vi "运维调试_氨氮.vi"() -> ()   [LabVIEW 2016, in "斯坦道氨氮.lvlib"]
uses:
  <vilib>/Utility/miscctls.llb/LVPointTypeDef.ctl
  <vilib>/Utility/config.llb/NI_LVConfig.lvlib
panel:
  in  "模块启用":bool
  in  "串口设置":bool
  in  "备用系数一键写入":bool
  in  "公式一键写入":bool
  in  "流程文件路径":path=path "C:/Users/std/Documents/斯坦道流程文件/流程.xml"
  in  "曲线模型":cluster{"X^2":dbl, "X":dbl, "B":dbl}(xcontrol)
  in  "质控参数设置":bool
  out "字符串":string
  in  "氨氮自动测试量程配置":T1
  out "ADC":sgl
  out "温度2":sgl
  out "温度1":sgl
  out "固件版本号":string
  in  "数组":string[](array[string])
  in  "备用系数写入":bool
  in  "备用系数读取":bool
  in  "备用系数":T2
  in  "量程切换阈值写入":bool
  in  "量程切换阈值读取":bool
  in  "量程切换阈值":cluster{"阈值":dbl, "标液浓度":dbl}
  in  "参数下拉列表":enum16{"氨氮", "总磷"}(ring)
  in  "量程下拉列表":enum16{"低量程", "高量程"}(ring)
  in  "测量模式下拉列表":enum16{"水样测量", "空白核查", "跨度核查", "标样核查", "加标回收"}(ring)
  in  "公式":cluster{"X^2":dbl, "X":dbl, "b":dbl}
  in  "写公式":bool
  in  "读公式":bool
  in  "返回":bool
  in  "设置":bool
  out "序列号":string="序列号"
  out "氨氮测量数据":T3(xcontrol)
  out "集成报警信息":string
  out "定时启动":bool
  out "总磷总氮运行状态":T4(xcontrol)
  in  "停止":bool
  in  "手动启动":bool
  in  "单步测试":bool
  in  "总磷氨氮调试":u16[](xcontrol)
  out "F3":sgl format="%#.6f"
  out "F2":sgl format="%#.6f"
  out "F1":sgl format="%#.6f"
  out "F0":sgl format="%#.6f"
  out "多列列表框":i32(listbox)
  # "参数设置"
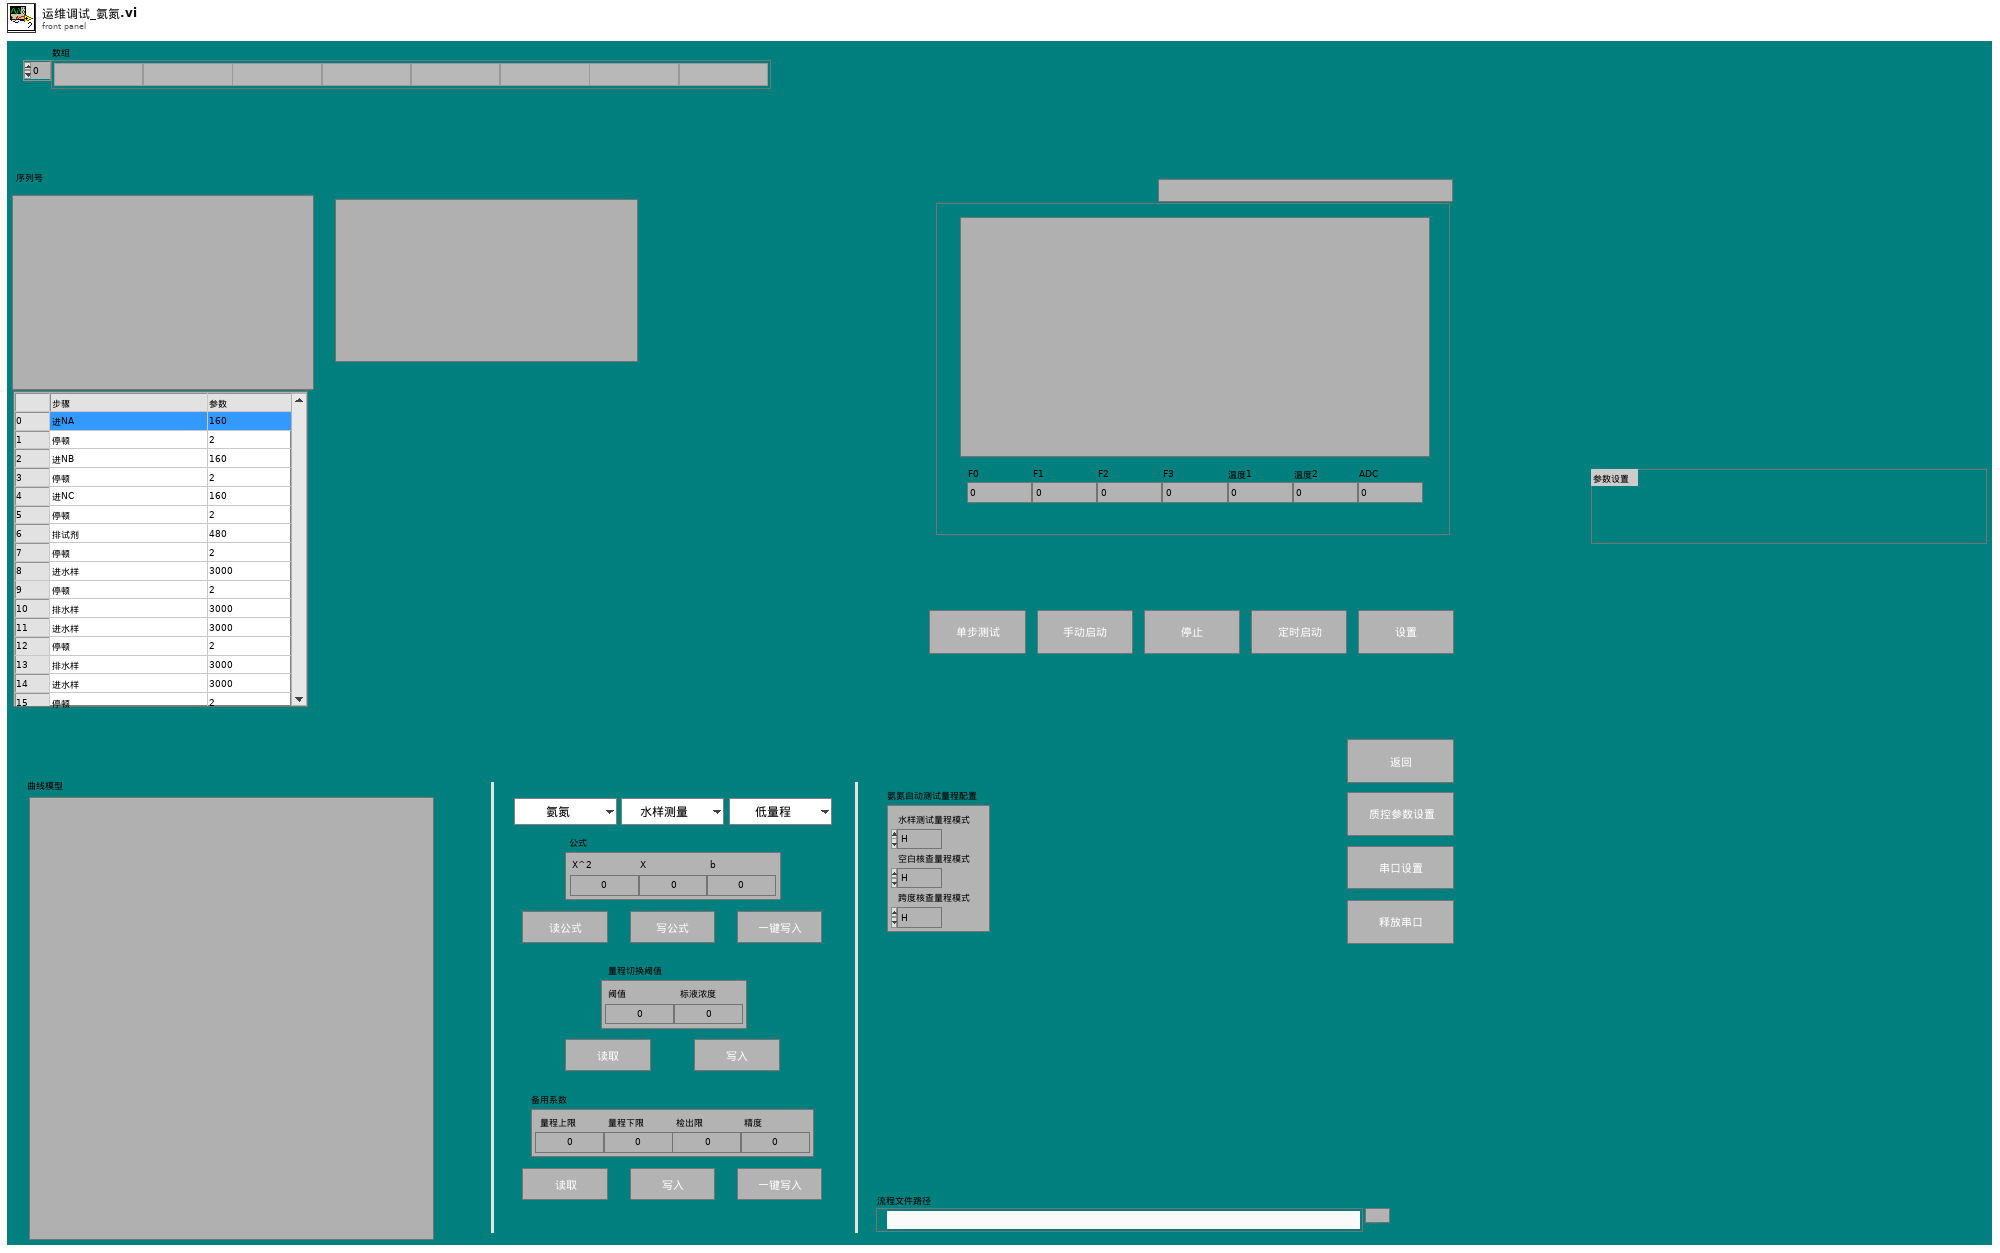
[diagram p1: front panel]
types:
  T1 = cluster{"水样测试量程模式":enum16{"H", "L", "AUTO"}, "空白核查量程模式":enum16{"H", "L", "AUTO"}, "跨度核查量程模式":enum16{"H", "L", "AUTO"}}
  T2 = cluster{"量程上限":dbl, "量程下限":dbl, "检出限":dbl, "精度":dbl}
  T3 = cluster{"flowid":u16, "测量精度":u16, "测量数据区":cluster{"因子编码":u32, "单位":u16, "标样参考值":sgl, "水样数据时间":timestamp, "水样实测值":sgl, "水样数据标识":string, "标样数据时间":timestamp, "标样实测值":sgl, "标样数据标识":string, "空白数据时间":timestamp, "空白实测值":sgl, "空白数据标识":string, "零点核查数据时间":timestamp, "零点核查实测值":sgl, "零点核查数据标识":string, "跨度核查数据时间":timestamp, "跨度核查实测值":sgl, "跨度核查数据标识":string, "加标回收数据时间":timestamp, "加标回收实测值":sgl, "加标回收数据标识":string, "平行样数据时间":timestamp, "平行样实测值":sgl, "平行样数据标识":string}}
  T4 = cluster{"系统时间":timestamp, "工作状态":enum16{"空闲", "水样测试", "标样核查", "零点核查", "跨度核查", "空白测试", "平行样测试", "加标回收", "空白校准", "标样校准", "初始化（清洗）"}, "测量模式":enum16{"待机", "连续模式", "周期模式", "定点模式", "受控模式", "手动模式"}, "告警代码":enum16{"无告警", "缺试剂告警", "缺水样告警", "缺蒸馏水告警", "缺标液告警", "仪表漏液告警", "标定异常告警", "超量程告警", "加热异常", "低试剂预警", "超上限告警", "超下限告警", "仪表内部其他异常", "滴定异常告警", "电极异常告警", "量程切换告警", "参数设置告警", "PH电极电位异常", "电导率电极异常", "浊度光度异常", "溶解氧电极异常", "溶解氧光强异常", "温度异常告警", "PH异常告警", "溶解氧异常告警", "电导率异常告警", "浊度异常告警", "叶绿素异常告警", "藻密度异常告警", "蓝绿藻异常告警", "ORP异常告警", "氨氮异常告警", "清洁刷异常告警", "SD卡异常告警", "蓝牙异常告警", "Wifi异常告警", "流程异常告警"}, "故障代码":enum16{"无故障", "电机故障", "温度故障", "通讯故障", "滴定故障"}, "日志代码":u16, "软件版本":u16, "F0":sgl, "F1":sgl, "F2":sgl, "F3":sgl, "T":sgl, "H":sgl, "id":u16, "flowid":u16, "量程":u16, "总磷控温温度1":sgl, "营养盐控温温度2":sgl, "ADC":sgl}
  T5 = enum16{"启动测量", "标样核查", "零点核查", "跨度核查", "空白测试", "平行样测试", "加标回收", "空白校准", "标样校准", "初始化（清洗）", "停止测试", "仪器重启", "校时", "模式设置", "测量间隔设置"}
  T6 = cluster{"控制命令":enum16{"启动测量", "标样核查", "零点核查", "跨度核查", "空白测试", "平行样测试", "加标回收", "空白校准", "标样校准", "初始化（清洗）", "停止测试", "仪器重启", "校时", "模式设置", "测量间隔设置"}, "周期设置类型":enum16{"定点启动", "间隔启动"}, "定时功能启用":bool, "定时间隔":dbl, "24H周期设置":bool[], "空白核查时间":u16, "跨度核查时间":u16, "质控频次":enum16{"关闭", "每天", "星期一", "星期二", "星期三", "星期四", "星期五", "星期六", "星期日"}}
  T7 = enum16{"关闭", "每天", "星期一", "星期二", "星期三", "星期四", "星期五", "星期六", "星期日"}
  T8 = enum32{"Bad", "Idle", "Run top level", "Running"}
  T9 = typedef "LVDateTimeRec.ctl" = cluster{"秒数的小数部分":dbl, "秒":i32, "分":i32, "时":i32, "日":i32, "月":i32, "年":i32, "天数（周）":i32, "天数（年）":i32, "DST":i32}
  T10 = typedef "LVPointTypeDef.ctl" = cluster{"Horizontal":i16, "Vertical":i16}
  T11 = cluster{"因子编码":u32, "单位":u16, "标样参考值":sgl, "水样数据时间":timestamp, "水样实测值":sgl, "水样数据标识":string, "标样数据时间":timestamp, "标样实测值":sgl, "标样数据标识":string, "空白数据时间":timestamp, "空白实测值":sgl, "空白数据标识":string, "零点核查数据时间":timestamp, "零点核查实测值":sgl, "零点核查数据标识":string, "跨度核查数据时间":timestamp, "跨度核查实测值":sgl, "跨度核查数据标识":string, "加标回收数据时间":timestamp, "加标回收实测值":sgl, "加标回收数据标识":string, "平行样数据时间":timestamp, "平行样实测值":sgl, "平行样数据标识":string}
  T12 = enum16{"空闲", "水样测试", "标样核查", "零点核查", "跨度核查", "空白测试", "平行样测试", "加标回收", "空白校准", "标样校准", "初始化（清洗）"}
  T13 = cluster{"启动模式":enum16{"跨度核查", "水样测量", "空白核查", "标样核查", "加标回收"}, "启动参数":u16, "量程":enum16{"低量程", "高量程"}}
  T14 = cluster{"时间标识":timestamp, "设备":string, "日志信息":string, "流程参数":string}
  T15 = cluster{"时间标识":timestamp, "设备":string, "日志信息":string}
  T16 = enum16{"无告警", "缺试剂告警", "缺水样告警", "缺蒸馏水告警", "缺标液告警", "仪表漏液告警", "标定异常告警", "超量程告警", "加热异常", "低试剂预警", "超上限告警", "超下限告警", "仪表内部其他异常", "滴定异常告警", "电极异常告警", "量程切换告警", "参数设置告警", "PH电极电位异常", "电导率电极异常", "浊度光度异常", "溶解氧电极异常", "溶解氧光强异常", "温度异常告警", "PH异常告警", "溶解氧异常告警", "电导率异常告警", "浊度异常告警", "叶绿素异常告警", "藻密度异常告警", "蓝绿藻异常告警", "ORP异常告警", "氨氮异常告警", "清洁刷异常告警", "SD卡异常告警", "蓝牙异常告警", "Wifi异常告警", "流程异常告警"}
  T17 = typedef "LVRowAndColumnUnsignedTypeDef.ctl" = cluster{"Row":u32, "Column":u32}
  T18 = typedef "NI_LVConfig.lvlib/Config Data RefNum.ctl" = refnum<k1>
  T19 = cluster{"站号":u16, "量程切换":enum32{"H", "L", "AUTO"}, "控制命令":enum16{"启动测量", "标样核查", "零点核查", "跨度核查", "空白测试", "平行样测试", "加标回收", "空白校准", "标样校准", "初始化（清洗）", "停止测试", "仪器重启", "校时", "模式设置", "测量间隔设置"}, "模式设置":enum16{"待机", "连续模式", "周期模式", "定点模式", "受控模式", "手动模式"}, "测量间隔":u16}
  T20 = cluster{"跨度值":dbl, "零点标准液浓度":dbl, "跨度标准液浓度":dbl, "标准液标准浓度":dbl}
  T21 = cluster{"确定":bool, "跨度值":dbl, "零点标准液浓度":dbl, "跨度标准液浓度":dbl, "标准液标准浓度":dbl}
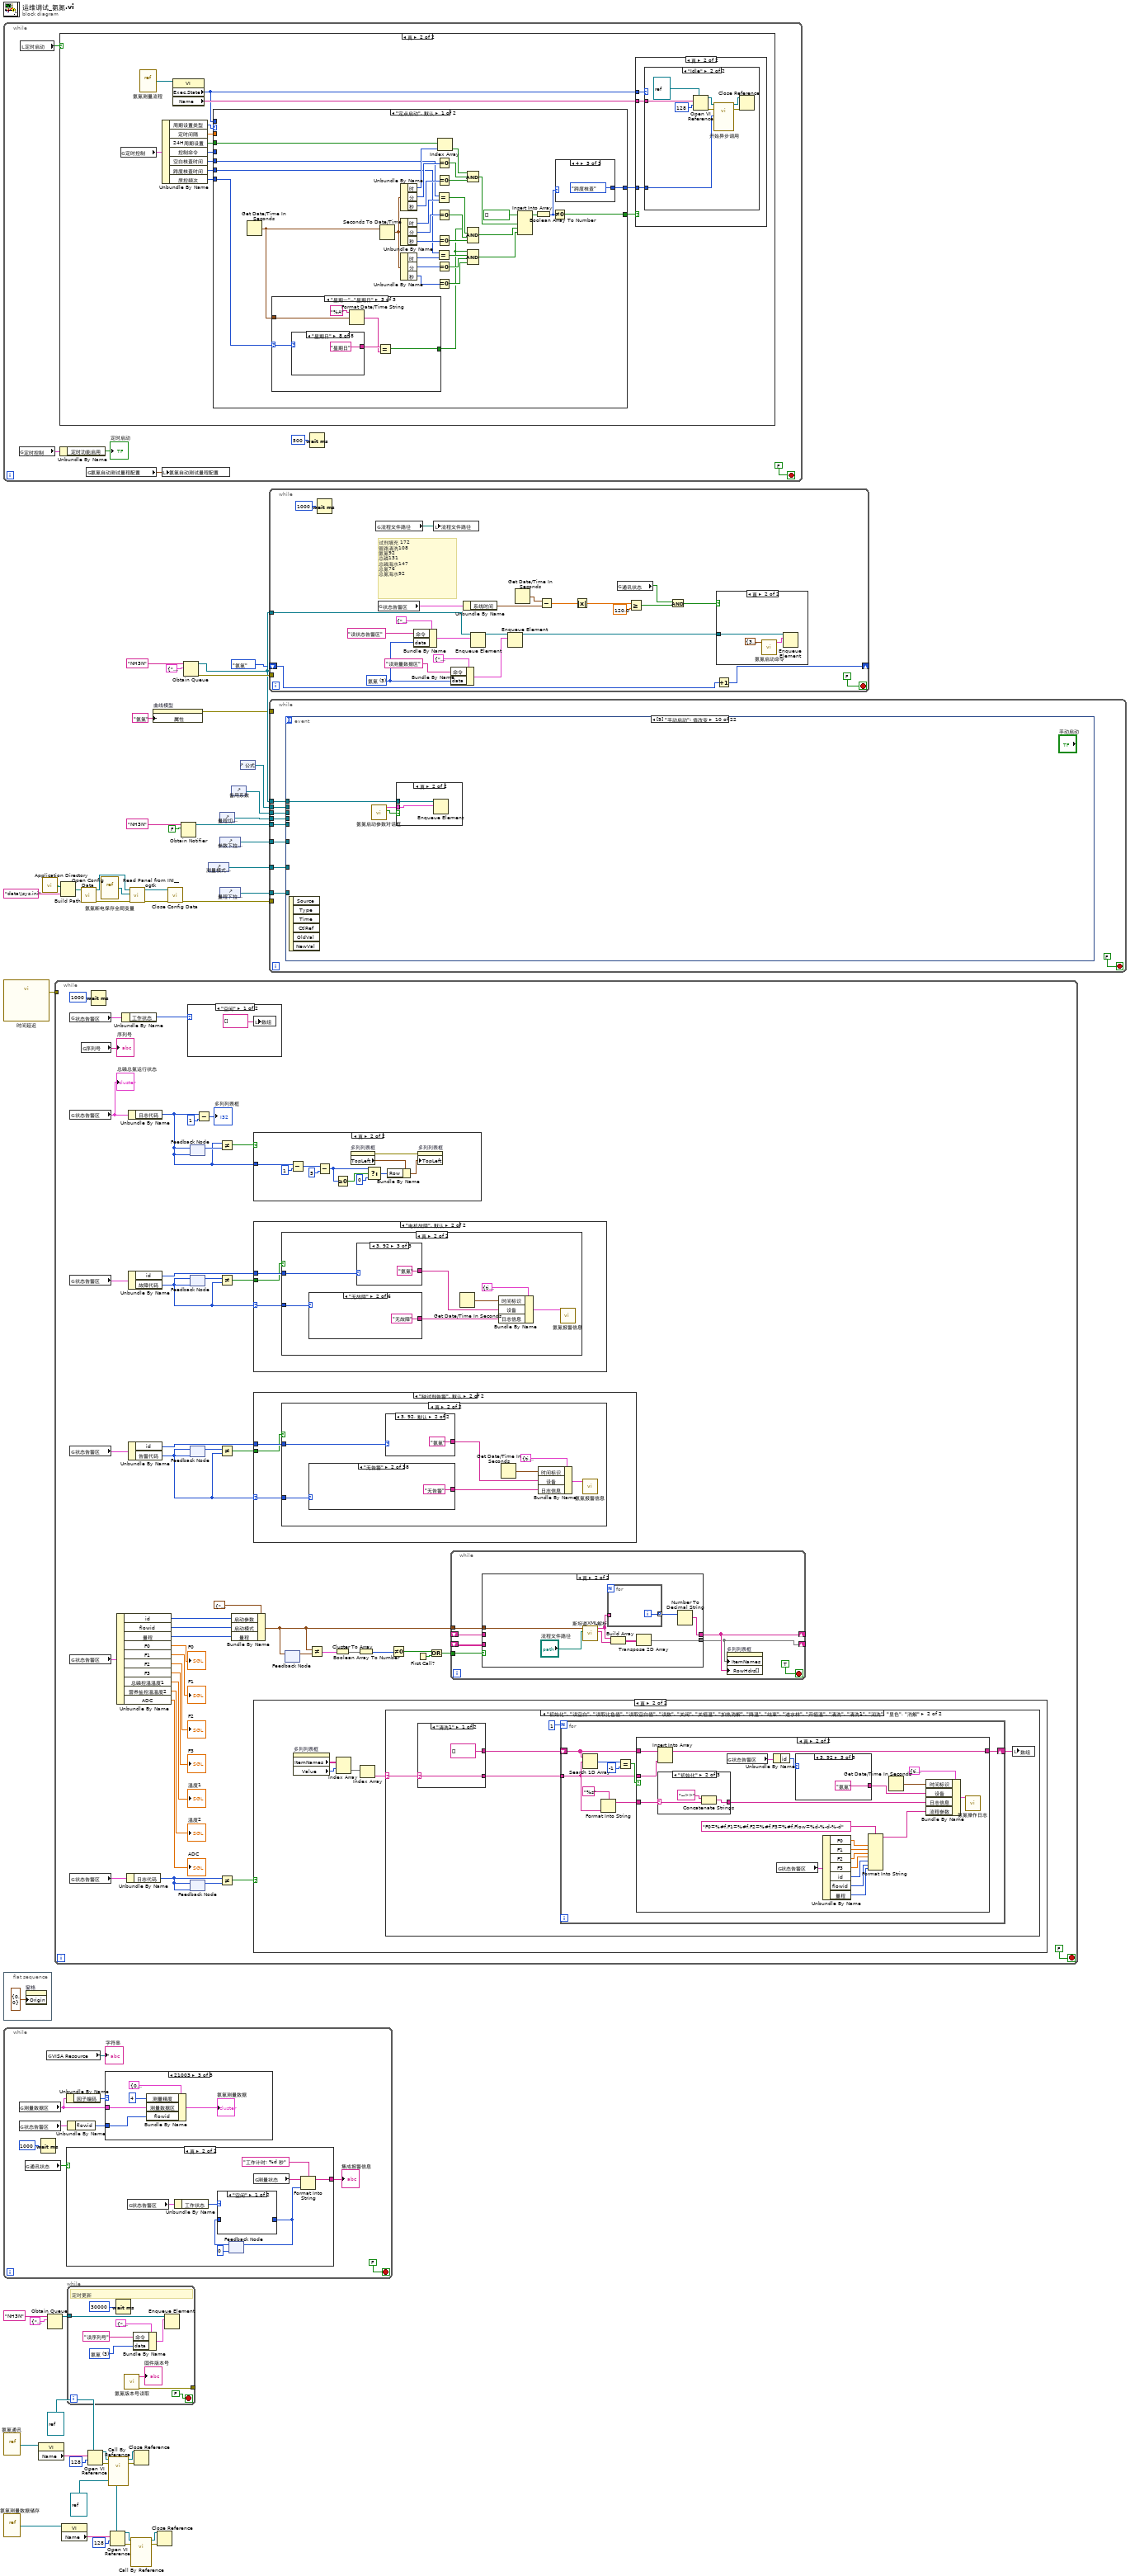
[diagram p0: block diagram]
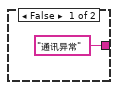
[diagram p2: hidden frame]
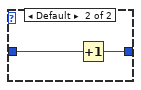
[diagram p3: hidden frame]
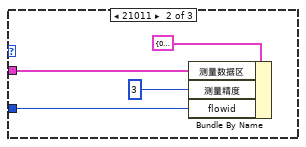
[diagram p5: hidden frame]
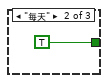
[diagram p8: hidden frame]
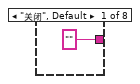
[diagram p9: hidden frame]
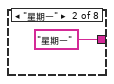
[diagram p10: hidden frame]
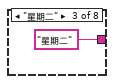
[diagram p11: hidden frame]
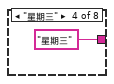
[diagram p12: hidden frame]
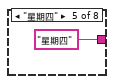
[diagram p13: hidden frame]
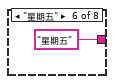
[diagram p14: hidden frame]
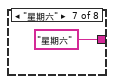
[diagram p15: hidden frame]
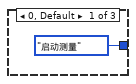
[diagram p16: hidden frame]
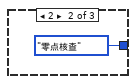
[diagram p17: hidden frame]
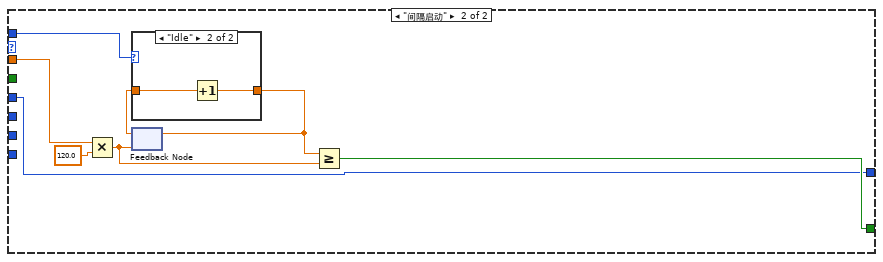
[diagram p18: hidden frame]
diagram:
  n1 = while {
    stop <- FALSE stop-if-true
    n2 = global read "氨氮断电保存全局变量.vi" "定时控制"() -> (w48:T6)
    n3 = local read "定时启动"() -> (w49:bool)
    n4 = case shown="真" w49 {
      frame False {
      }
      frame True {
        n5 = global read "氨氮断电保存全局变量.vi" "定时控制"() -> (w64:T6)
        n6 = vi-ref "氨氮测量流程.vi"() -> (w63:refnum<vi>)
        n7 = Unbundle By Name(w64) -> ("周期设置类型"=w60:enum16{"定点启动", "间隔启动"}, "定时间隔"=w59:dbl, "24H周期设置"=w58:bool[], "控制命令"=w57:T5, "空白核查时间"=w54:u16, "跨度核查时间"=w53:u16, "质控频次"=w52:T7)
        n8 = property class="VI"(reference=w63) -> ("Exec.State"=w61:T8, "Name"=w62:string)  [unwired: 1 in, 2 out]
        n9 = case shown="\"定点启动\", 默认" w60 {
          tunnel: w59 -> [_ w120]
          tunnel: w58 -> [w88 _]
          tunnel: w61 -> [_ w123]
          tunnel: [w66 w118] -> w55
          tunnel: w57 -> [_ w116]
          tunnel: [w92 w116] -> w56
          tunnel: w52 -> [w91 _]
          tunnel: w54 -> [w84 _]
          tunnel: w53 -> [w73 _]
          frame "定点启动", Default {
            n10 = Get Date/Time In Seconds() -> (seconds since 1Jan1904=w90:timestamp)
            n11 = case shown="\"星期一\"..\"星期日\"" w91 {
              selector: w91 -> [_ _ w102]
              tunnel: w90 -> [_ _ w103]
              tunnel: [_ TRUE w99] -> w72
              frame "关闭", Default {
              }
              frame "每天" {
              }
              frame "星期一".."星期日" {
                n12 = case shown="\"星期日\"" w102 {
                  tunnel: ["" ("时间格式字符串(%c)") "星期一" ("时间格式字符串(%c)") "星期二" ("时间格式字符串(%c)") "星期三" ("时间格式字符串(%c)") "星期四" ("时间格式字符串(%c)") "星期五" ("时间格式字符串(%c)") "星期六" ("时间格式字符串(%c)") "星期日" ("时间格式字符串(%c)")] -> w101
                  frame "关闭", Default {
                  }
                  frame "星期一" {
                  }
                  frame "星期二" {
                  }
                  frame "星期三" {
                  }
                  frame "星期四" {
                  }
                  frame "星期五" {
                  }
                  frame "星期六" {
                  }
                  frame "星期日" {
                  }
                }
                n13 = Format Date/Time String(time format string (%c)="%A" ("时间格式字符串(%c)"), seconds (now)=w103) -> (date/time string=w100:string)  [unwired: 1 in]
                n14 = Equal?(x=w101, y=w100) -> (x = y?=w99:bool)
              }
            }
            n15 = Seconds To Date/Time(time stamp (now)=w90) -> (date time rec=w74:T9)  [unwired: 1 in]
            n16 = Unbundle By Name(w74) -> ("时"=w97:i32, "分"=w95:i32, "秒"=w96:i32)
            n17 = Unbundle By Name(w74) -> ("时"=w85:i32, "分"=w87:i32, "秒"=w86:i32)
            n18 = Unbundle By Name(w74) -> ("时"=w77:i32, "分"=w75:i32, "秒"=w76:i32)
            n19 = Equal?(x=w84, y=w85) -> (x = y?=w83:bool)
            n20 = Equal?(x=w73, y=w77) -> (x = y?=w78:bool)
            n21 = Equal To 0?(x=w95) -> (x = 0?=w94:bool)
            n22 = Equal To 0?(x=w96) -> (x = 0?=w93:bool)
            n23 = Equal To 0?(x=w87) -> (x = 0?=w82:bool)
            n24 = Equal To 0?(x=w86) -> (x = 0?=w81:bool)
            n25 = Equal To 0?(x=w75) -> (x = 0?=w79:bool)
            n26 = Equal To 0?(x=w76) -> (x = 0?=w80:bool)
            n27 = Index Array(array=w88, index=w97) -> (element=w89:bool)
            n28 = Compound Arithmetic op=AND ("复合运算")(w89, w94, w93) -> (w70:bool)
            n29 = Compound Arithmetic op=AND ("复合运算")(w72, w83, w82, w81) -> (w69:bool)
            n30 = Compound Arithmetic op=AND ("复合运算")(w72, w78, w79, w80) -> (w68:bool)
            n31 = Insert Into Array(array=bool[] [], new element #1=w70, new element #2=w69, new element #3=w68) -> (w67:bool[])  [unwired: 1 in]
            n32 = Boolean Array To Number(Boolean array=w67) -> (number=w65:u32)
            n33 = Not Equal To 0?(x=w65) -> (x != 0?=w66:bool)
            n34 = case shown="4" w65 {
              tunnel: [T5."启动测量" ("控制命令") T5."零点核查" ("控制命令") T5."跨度核查" ("控制命令")] -> w92
              frame 0, Default {
              }
              frame 2 {
              }
              frame 4 {
              }
            }
          }
          frame "间隔启动" {
            n35 = Multiply(x=w120, y=120.0) -> (x*y=w117:dbl)
            n36 = feedback #1(w117) -> (w122:dbl)
            n37 = case shown="\"Idle\"" w123 {
              tunnel: w122 -> [_ w125]
              tunnel: [_ w124] -> w121
              frame "Bad", Default {
              }
              frame "Idle" {
                n38 = Increment(x=w125) -> (x+1=w124:dbl)
              }
            }
            n39 = feedback-in #1(w121) -> ()
            n40 = Greater Or Equal?(x=w121, y=w117) -> (x >= y?=w118:bool)
          }
        }
        n41 = case shown="真" w55 {
          tunnel: w62 -> [_ w128]
          tunnel: w56 -> [_ w127]
          tunnel: w61 -> [_ w126]
          frame False {
          }
          frame True {
            n42 = case shown="\"Idle\"" w126 {
              tunnel: w128 -> [_ w132]
              tunnel: w127 -> [_ w130]
              frame "Bad", Default {
              }
              frame "Idle" {
                n43 = Open VI Reference(type specifier VI Refnum (for type only)=refnum<vi> refnum, vi path=w132, options=128 ("选项")) -> (vi reference=w133:refnum<vi>, error out=w134:errorcluster)  [unwired: 3 in]
                n44 = call-by-ref "开始异步调用"(reference=w133, error in=w134, "控制命令"=w130) -> (reference out=w135:refnum<vi>, error out=w136:errorcluster)  [unwired: 11 in]
                n45 = Close Reference(reference=w135, error in (no error)=w136) -> ()  [unwired: 1 out]
              }
            }
          }
        }
      }
    }
    n46 = Unbundle By Name(w48) -> ("定时功能启用"=→"定时启动":bool)
    n47 = global read "氨氮断电保存全局变量.vi" "氨氮自动测试量程配置"() -> (w46:T1)
    n48 = local write "氨氮自动测试量程配置"(w46) -> ()
    n49 = Wait (ms)(milliseconds to wait=u32 500 ("等待时间（毫秒）")) -> ()  [unwired: 1 out]
  }
  n50 = call "时间延迟"() -> ("error out"=w18:errorcluster)  [unwired: 11 in]
  n51 = flat-sequence {
    frame #0 {
      n52 = property on="窗格" class="Pane"("Origin"=T10 {"Horizontal"=0, "Vertical"=0} ("原点")) -> ()  [unwired: 2 in, 2 out]
    }
  }
  n53 = while {
    stop <- FALSE stop-if-true
    n54 = global read "VAR氨氮全局变量.vi" "测量数据区"() -> (w144:T11)
    n55 = global read "VAR氨氮全局变量.vi" "状态告警区"() -> (w140:T4)
    n56 = global read "VAR氨氮全局变量.vi" "通讯状态"() -> (w142:bool)
    n57 = Wait (ms)(milliseconds to wait=u32 1000 ("等待时间（毫秒）")) -> ()  [unwired: 1 out]
    n58 = global read "氨氮断电保存全局变量.vi" "VISA Resource"() -> (→"字符串":refnum<visa-resource-name>)
    n59 = Unbundle By Name(w144) -> ("因子编码"=w143:u32)
    n60 = case shown="真" w142 {
      tunnel: ["通讯异常" ("集成报警信息") w149] -> w141
      frame False {
      }
      frame True {
        n61 = global read "VAR氨氮全局变量.vi" "状态告警区"() -> (w155:T4)
        n62 = Unbundle By Name(w155) -> ("工作状态"=w154:T12)
        n63 = feedback #2(0) -> (w152:i32)
        n64 = case shown="\"空闲\"" w154 {
          tunnel: w152 -> [_ w157]
          tunnel: [_ w156] -> w150
          frame "空闲" {
          }
          frame Default {
            n65 = Increment(x=w157) -> (x+1=w156:i32)
          }
        }
        n66 = feedback-in #2(w150) -> ()
        n67 = global read "VAR氨氮全局变量.vi" "测量状态"() -> (w148:string)
        n68 = Format Into String(format string="工作计时: %d 秒" ("格式字符串"), initial string=w148, w150) -> (resulting string=w149:string)  [unwired: 1 in, 1 out]
      }
    }
    "集成报警信息" <- w141
    n69 = Unbundle By Name(w140) -> ("flowid"=w139:u16)
    n70 = case shown="21003" w143 {
      tunnel: w144 -> [_ w161 w166]
      tunnel: w139 -> [_ w159 w164]
      frame Default {
      }
      frame 21011 {
        n71 = Bundle By Name(cluster=T3 {"flowid"=0, "测量精度"=0, "测量数据区"={"因子编码"=0, "单位"=0, "标样参考值"=0.0, "水样数据时间"=timestamp(0 s since 1904-01-01), "水样实测值"=0.0, "水样数据标识"="", "标样数据时间"=timestamp(0 s since 1904-01-01), "标样实测值"=0.0, "标样数据标识"="", "空白数据时间"=timestamp(0 s since 1904-01-01), "空白实测值"=0.0, "空白数据标识"="", "零点核查数据时间"=timestamp(0 s since 1904-01-01), "零点核查实测值"=0.0, "零点核查数据标识"="", "跨度核查数据时间"=timestamp(0 s since 1904-01-01), "跨度核查实测值"=0.0, "跨度核查数据标识"="", "加标回收数据时间"=timestamp(0 s since 1904-01-01), "加标回收实测值"=0.0, "加标回收数据标识"="", "平行样数据时间"=timestamp(0 s since 1904-01-01), "平行样实测值"=0.0, "平行样数据标识"=""}} ("氨氮测量数据"), "测量数据区"=w161, "测量精度"=u16 3, "flowid"=w159) -> ()  [unwired: 1 out]
      }
      frame 21003 {
        n72 = Bundle By Name(cluster=T3 {"flowid"=0, "测量精度"=0, "测量数据区"={"因子编码"=0, "单位"=0, "标样参考值"=0.0, "水样数据时间"=timestamp(0 s since 1904-01-01), "水样实测值"=0.0, "水样数据标识"="", "标样数据时间"=timestamp(0 s since 1904-01-01), "标样实测值"=0.0, "标样数据标识"="", "空白数据时间"=timestamp(0 s since 1904-01-01), "空白实测值"=0.0, "空白数据标识"="", "零点核查数据时间"=timestamp(0 s since 1904-01-01), "零点核查实测值"=0.0, "零点核查数据标识"="", "跨度核查数据时间"=timestamp(0 s since 1904-01-01), "跨度核查实测值"=0.0, "跨度核查数据标识"="", "加标回收数据时间"=timestamp(0 s since 1904-01-01), "加标回收实测值"=0.0, "加标回收数据标识"="", "平行样数据时间"=timestamp(0 s since 1904-01-01), "平行样实测值"=0.0, "平行样数据标识"=""}} ("氨氮测量数据"), "测量精度"=u16 4, "测量数据区"=w166, "flowid"=w164) -> (→"氨氮测量数据":T3)
      }
    }
  }
  n73 = vi-ref "氨氮通讯.vi"() -> (w41:refnum<vi>)
  n74 = vi-ref "氨氮测量数据储存.vi"() -> (w33:refnum<vi>)
  n75 = property class="VI"(reference=w41) -> ("Name"=w40:string)  [unwired: 1 in, 2 out]
  n76 = call <vilib>:"Application Directory.vi"() -> ("Application Directory"=w4:path)
  n77 = Obtain Queue(name (unnamed)="NH3N" ("名称（未命名）"), element data type=cluster{"命令":string, "data":variant} {"命令"="", "data"=variant}) -> (queue out=w15:refnum<queue>)  [unwired: 3 in, 2 out]
  n78 = while {
    tunnel: w18 -> [_]
    stop <- FALSE stop-if-true
    n79 = global read "VAR氨氮全局变量.vi" "状态告警区"() -> (w179:T4)
    n80 = global read "VAR氨氮全局变量.vi" "状态告警区"() -> (w192:T4)
    "总磷总氮运行状态" <- w192
    n81 = global read "VAR氨氮全局变量.vi" "状态告警区"() -> (w184:T4)
    n82 = global read "VAR氨氮全局变量.vi" "状态告警区"() -> (w189:T4)
    n83 = global read "VAR氨氮全局变量.vi" "状态告警区"() -> (w200:T4)
    n84 = global read "VAR氨氮全局变量.vi" "状态告警区"() -> (w176:T4)
    n85 = global read "VAR氨氮全局变量.vi" "序列号"() -> (→"序列号":string)
    n86 = Wait (ms)(milliseconds to wait=u32 1000 ("等待时间（毫秒）")) -> ()  [unwired: 1 out]
    n87 = Unbundle By Name(w200) -> ("id"=w197:u16, "flowid"=w199:u16, "量程"=w198:u16, "F0"=→"F0":sgl, "F1"=→"F1":sgl, "F2"=→"F2":sgl, "F3"=→"F3":sgl, "总磷控温温度1"=→"温度1":sgl, "营养盐控温温度2"=→"温度2":sgl, "ADC"=→"ADC":sgl)
    n88 = Unbundle By Name(w179) -> ("工作状态"=w178:T12)
    n89 = Unbundle By Name(w176) -> ("日志代码"=w175:u16)
    n90 = Unbundle By Name(w192) -> ("日志代码"=w169:u16)
    n91 = Unbundle By Name(w184) -> ("id"=w183:u16, "故障代码"=w180:enum16{"无故障", "电机故障", "温度故障", "通讯故障", "滴定故障"})
    n92 = Unbundle By Name(w189) -> ("id"=w188:u16, "告警代码"=w185:T16)
    n93 = case shown="\"空闲\"" w178 {
      frame "空闲" {
        n94 = local write "数组"(string[] [] ("数组")) -> ()
      }
      frame "水样测试", Default {
      }
    }
    n95 = feedback-in #3(w169) -> ()
    n96 = feedback #3(w169) -> (w209:u16)
    n97 = feedback #4(w180) -> (w181:enum16{"无故障", "电机故障", "温度故障", "通讯故障", "滴定故障"})
    n98 = feedback-in #4(w180) -> ()
    n99 = feedback #5(w185) -> (w186:T16)
    n100 = feedback-in #5(w185) -> ()
    n101 = feedback #6(w175) -> (w177:u16)
    n102 = feedback-in #6(w175) -> ()
    n103 = Subtract(x=w169, y=1) -> (x-y=→"多列列表框":i32)
    n104 = Not Equal?(x=w169, y=w209) -> (x != y?=w208:bool)
    n105 = Not Equal?(x=w181, y=w180) -> (x != y?=w182:bool)
    n106 = Not Equal?(x=w186, y=w185) -> (x != y?=w187:bool)
    n107 = Not Equal?(x=w175, y=w177) -> (x != y?=w174:bool)
    n108 = Bundle By Name(cluster=T13 {"启动模式"=enum."跨度核查", "启动参数"=1, "量程"=enum."低量程"} ("参数簇"), "启动参数"=w197, "启动模式"=w199, "量程"=w198) -> (w191:T13)
    n109 = case shown="真" w208 {
      tunnel: w169 -> [_ w359]
      frame False {
      }
      frame True {
        n110 = Subtract(x=w359, y=1) -> (x-y=w357:i32)
        n111 = Subtract(x=w357, y=5) -> (x-y=w361:i32)
        n112 = Greater Or Equal To 0?(x=w361) -> (x >= 0?=w360:bool)
        n113 = property on="多列列表框" class="MCListbox (严格)"() -> (error out=w365:errorcluster, "TopLeft"=w366:T17)  [unwired: 2 in, 1 out]
        n114 = Select(t=w361, s=w360, f=0) -> (s? t:f=w362:i32)
        n115 = Bundle By Name(cluster=w366, "Row"=w362) -> (w367:T17)
        n116 = property on="多列列表框" class="MCListbox (严格)"(error in=w365, "TopLeft"=w367) -> ()  [unwired: 1 in, 2 out]
      }
    }
    n117 = case shown="\"电机故障\", 默认" w180 {
      selector: w180 -> [_ w266]
      tunnel: w183 -> [_ w267]
      tunnel: w182 -> [_ w265]
      frame "无故障" {
      }
      frame "电机故障", Default {
        n118 = case shown="真" w265 {
          tunnel: w267 -> [_ w274]
          tunnel: w266 -> [_ w269]
          frame False {
          }
          frame True {
            n119 = case shown="\"无故障\"" w269 {
              selector: w269 -> [w276 _ _ _ _ _]
              tunnel: [w275 "无故障" "电机故障" "温度故障" "通讯故障" "滴定故障"] -> w268
              frame Default {
                n120 = Format Into String(format string="%d" ("格式字符串"), initial string="未知" ("工作状态"), w276) -> (resulting string=w275:string)  [unwired: 1 in, 1 out]
              }
              frame "无故障" {
              }
              frame "电机故障" {
              }
              frame "温度故障" {
              }
              frame "通讯故障" {
              }
              frame "滴定故障" {
              }
            }
            n121 = case shown="3, 92" w274 {
              tunnel: [_ "总磷" ("table输入") "氨氮" ("table输入")] -> w270
              frame Default {
              }
              frame 1, 131 {
              }
              frame 3, 92 {
              }
            }
            n122 = Get Date/Time In Seconds() -> (seconds since 1Jan1904=w271:timestamp)
            n123 = Bundle By Name(cluster=T15 {"时间标识"=timestamp(0 s since 1904-01-01), "设备"="", "日志信息"=""} ("data in"), "时间标识"=w271, "设备"=w270, "日志信息"=w268) -> (w272:T15)
            n124 = call "氨氮报警信息.vi"("data in"=w272) -> ()  [unwired: 11 in]
          }
        }
      }
    }
    n125 = case shown="\"缺试剂告警\", 默认" w185 {
      selector: w185 -> [_ w287]
      tunnel: w188 -> [_ w288]
      tunnel: w187 -> [_ w286]
      frame "无告警" {
      }
      frame "缺试剂告警", Default {
        n126 = case shown="真" w286 {
          tunnel: w288 -> [_ w295]
          tunnel: w287 -> [_ w289]
          frame False {
          }
          frame True {
            n127 = case shown="\"无告警\"" w289 {
              selector: w289 -> [w297 _ _ _ _ _ _ _ _ _ _ _ _ _ _ _ _ _ _ _ _ _ _ _ _ _ _ _ _ _ _ _ _ _ _ _ _ _]
              tunnel: [w296 "无告警" "缺试剂告警" "缺水样告警" "缺蒸馏水告警" "缺标液告警" "仪表漏液告警" "标定异常告警" "超量程告警" "加热异常" "低试剂预警" "超上限告警" "超下限告警" "仪表内部其他异常" "滴定异常告警" "电极异常告警" "量程切换告警" "参数设置告警" "PH电极电位异常" "电导率电极异常" "浊度光度异常" "溶解氧电极异常" "溶解氧光强异常" "温度异常告警" "PH异常告警" "溶解氧异常告警" "电导率异常告警" "浊度异常告警" "叶绿素异常告警" "藻密度异常告警" "蓝绿藻异常告警" "ORP异常告警" "氨氮异常告警" "清洁刷异常告警" "SD卡异常告警" "蓝牙异常告警" "WiFi异常告警" "流程异常告警"] -> w290
              frame Default {
                n128 = Format Into String(format string="%d" ("格式字符串"), initial string="未知" ("工作状态"), w297) -> (resulting string=w296:string)  [unwired: 1 in, 1 out]
              }
              frame "无告警" {
              }
              frame "缺试剂告警" {
              }
              frame "缺水样告警" {
              }
              frame "缺蒸馏水告警" {
              }
              frame "缺标液告警" {
              }
              frame "仪表漏液告警" {
              }
              frame "标定异常告警" {
              }
              frame "超量程告警" {
              }
              frame "加热异常" {
              }
              frame "低试剂预警" {
              }
              frame "超上限告警" {
              }
              frame "超下限告警" {
              }
              frame "仪表内部其他异常" {
              }
              frame "滴定异常告警" {
              }
              frame "电极异常告警" {
              }
              frame "量程切换告警" {
              }
              frame "参数设置告警" {
              }
              frame "PH电极电位异常" {
              }
              frame "电导率电极异常" {
              }
              frame "浊度光度异常" {
              }
              frame "溶解氧电极异常" {
              }
              frame "溶解氧光强异常" {
              }
              frame "温度异常告警" {
              }
              frame "PH异常告警" {
              }
              frame "溶解氧异常告警" {
              }
              frame "电导率异常告警" {
              }
              frame "浊度异常告警" {
              }
              frame "叶绿素异常告警" {
              }
              frame "藻密度异常告警" {
              }
              frame "蓝绿藻异常告警" {
              }
              frame "ORP异常告警" {
              }
              frame "氨氮异常告警" {
              }
              frame "清洁刷异常告警" {
              }
              frame "SD卡异常告警" {
              }
              frame "蓝牙异常告警" {
              }
              frame "Wifi异常告警" {
              }
              frame "流程异常告警" {
              }
            }
            n129 = case shown="3, 92, 默认" w295 {
              tunnel: ["总磷" ("table输入") "氨氮" ("table输入")] -> w291
              frame 1, 131 {
              }
              frame 3, 92, Default {
              }
            }
            n130 = Get Date/Time In Seconds() -> (seconds since 1Jan1904=w292:timestamp)
            n131 = Bundle By Name(cluster=T15 {"时间标识"=timestamp(0 s since 1904-01-01), "设备"="", "日志信息"=""} ("data in"), "时间标识"=w292, "设备"=w291, "日志信息"=w290) -> (w293:T15)
            n132 = call "氨氮报警信息.vi"("data in"=w293) -> ()  [unwired: 11 in]
          }
        }
      }
    }
    n133 = case shown="真" w174 {
      frame False {
      }
      frame True {
        n134 = property on="多列列表框" class="MCListbox (严格)"() -> ("ItemNames"=w215:string[][], "Value"=w216:i32)  [unwired: 2 in, 2 out]
        n135 = Index Array(array=w215, index (row)=w216) -> (element=w214:string[])  [unwired: 1 in]
        n136 = Index Array(array=w214) -> (element=w213:string)  [unwired: 1 in]
        n137 = case shown="\"初始化\", \"读空白\", \"读取比色值\", \"读取空白值\", \"读数\", \"关阀\", \"关恒温\", \"加热消解\", \"降温\", \"结束\", \"进水样\", \"开恒温\", \"清洗\", \"清洗1\", \"润洗\", \"显色\", \"消解\"" w213 {
          selector: w213 -> [_ w219]
          frame Default {
          }
          frame "初始化", "读空白", "读取比色值", "读取空白值", "读数", "关阀", "关恒温", "加热消解", "降温", "结束", "进水样", "开恒温", "清洗", "清洗1", "润洗", "显色", "消解" {
            n138 = case shown="\"清洗1\"" w219 {
              selector: w219 -> [w223 w225]
              tunnel: [w223 w225] -> w218
              tunnel: [string[] [] ("数组") "数组"] -> w217
              frame "清洗1" {
              }
              frame Default {
              }
            }
            n139 = for {
              N: 1 -> [_]
              tunnel: w218 -> [w227]
              shift-right: [w226] -> w220
              shift-left: w217 -> [w228]
              n140 = Search 1D Array(1D array=w228, element=w227) -> (index of element=w231:i32)  [unwired: 1 in]
              n141 = Format Into String(format string="%s" ("格式字符串"), w227) -> (resulting string=w232:string)  [unwired: 2 in, 1 out]
              n142 = Equal?(x=w231, y=-1) -> (x = y?=w229:bool)
              n143 = case shown="真" w229 {
                tunnel: w232 -> [_ w236]
                tunnel: w228 -> [w234 w240]
                tunnel: w227 -> [_ w239]
                tunnel: [w234 w238] -> w226
                frame False {
                }
                frame True {
                  n144 = Insert Into Array(array=w240, new element=w239) -> (w238:string[])  [unwired: 1 in]
                  n145 = case shown="\"初始化\"" w236 {
                    selector: w236 -> [w256 w259 w262]
                    tunnel: [w256 w258 w261] -> w235
                    frame Default {
                    }
                    frame "初始化" {
                      n146 = Concatenate Strings("-->>" ("字符串"), w259) -> (w258:string)
                    }
                    frame "结束" {
                      n147 = Concatenate Strings("-->>" ("字符串"), w262) -> (w261:string)
                    }
                  }
                  n148 = global read "VAR氨氮全局变量.vi" "状态告警区"() -> (w255:T4)
                  n149 = Unbundle By Name(w255) -> ("id"=w254:u16)
                  n150 = global read "VAR氨氮全局变量.vi" "状态告警区"() -> (w250:T4)
                  n151 = case shown="3, 92" w254 {
                    tunnel: [_ "总磷" ("table输入") "氨氮" ("table输入")] -> w252
                    frame Default {
                    }
                    frame 1, 131 {
                    }
                    frame 3, 92 {
                    }
                  }
                  n152 = Unbundle By Name(w250) -> ("F0"=w247:sgl, "F1"=w246:sgl, "F2"=w245:sgl, "F3"=w244:sgl, "id"=w243:u16, "flowid"=w242:u16, "量程"=w241:u16)
                  n153 = Format Into String(format string="F0=%#f,F1=%#f,F2=%#f,F3=%#f,Flow=%d-%-d-%-d" ("格式字符串"), w247, w246, w245, w244, w243, w242, w241) -> (resulting string=w248:string)  [unwired: 2 in, 1 out]
                  n154 = Get Date/Time In Seconds() -> (seconds since 1Jan1904=w251:timestamp)
                  n155 = Bundle By Name(cluster=T14 {"时间标识"=timestamp(0 s since 1904-01-01), "设备"="", "日志信息"="", "流程参数"=""} ("data in"), "时间标识"=w251, "设备"=w252, "日志信息"=w235, "流程参数"=w248) -> (w253:T14)
                  n156 = call "氨氮操作日志.vi"("data in"=w253) -> ()  [unwired: 11 in]
                }
              }
            }
            n157 = local write "数组"(w220) -> ()
          }
        }
      }
    }
    n158 = feedback #7() -> (w204:T13)  [unwired: 1 in]
    n159 = feedback-in #7(w191) -> ()
    n160 = Not Equal?(x=w191, y=w204) -> (x != y?=w205:cluster{"启动模式":bool, "启动参数":bool, "量程":bool})
    n161 = Cluster To Array(cluster=w205) -> (array=w206:bool[])
    n162 = Boolean Array To Number(Boolean array=w206) -> (number=w207:u32)
    n163 = Not Equal To 0?(x=w207) -> (x != 0?=w202:bool)
    n164 = First Call?() -> (First Call?: T/F=w203:bool)
    n165 = Or(x=w202, y=w203) -> (x .or. y?=w201:bool)
    n166 = while {
      tunnel: w201 -> [w345]
      tunnel: w191 -> [w344]
      shift-right: [w339] -> _
      shift-left: _ -> [w341]
      shift-right: [w340] -> _
      shift-left: _ -> [w342]
      stop <- TRUE stop-if-true
      n167 = case shown="真" w345 {
        tunnel: [w347 w355] -> w340
        tunnel: [w346 w354] -> w339
        tunnel: w344 -> [_ w349]
        tunnel: w342 -> [w347 _]
        tunnel: w341 -> [w346 _]
        frame False {
        }
        frame True {
          n168 = call "斯坦道XML解析.vi"("添加的路径"="流程文件路径", "参数簇"=w349) -> ("步骤时间"=w350:string[], "步骤名"=w352:string[])  [unwired: 8 in]
          n169 = for {
            tunnel: w352 -> [_] mode=indexing
            tunnel: [w356] -> w353 mode=indexing
            i -> [w356]
          }
          n170 = Build Array(w352, w350) -> (w351:string[][])
          n171 = Transpose 2D Array(2D array=w351) -> (transposed array=w354:string[][])
          n172 = Number To Decimal String(number=w353) -> (decimal integer string=w355:string[])  [unwired: 1 in]
        }
      }
      n173 = property on="多列列表框" class="MCListbox (严格)"("ItemNames"=w339, "RowHdrs[]"=w340) -> ()  [unwired: 2 in, 2 out]
    }
  }
  n174 = Build Path(base path=w4, name or relative path="data\\sys.ini" ("名称或相对路径")) -> (appended path=w6:path)
  n175 = property class="VI"(reference=w33) -> ("Name"=w26:string)  [unwired: 1 in, 2 out]
  n176 = while {
    tunnel: w15 -> [w372]
    tunnel: [w369] -> _
    stop <- FALSE stop-if-true
    w373 = u16 3 items=["总磷"=1, "氨氮"=3] ("站号")
    # "定时更新"
    n177 = Wait (ms)(milliseconds to wait=u32 30000 ("等待时间（毫秒）")) -> ()  [unwired: 1 out]
    n178 = call "氨氮版本号读取.vi"() -> ("error out"=w369:errorcluster, "固件版本号"=→"固件版本号":string)  [unwired: 10 in]
    n179 = Bundle By Name(cluster=cluster{"命令":string, "data":variant} {"命令"="", "data"=variant} ("元素"), "命令"="读序列号", "data"=w373) -> (w371:cluster{"命令":string, "data":variant})
    n180 = Enqueue Element(queue=w372, element=w371) -> ()  [unwired: 2 in, 3 out]
  }
  n181 = call <vilib>:"Open Config Data.vi"("configuration file path"=w6) -> ("error out"=w10:errorcluster, "refnum"=w7:T18)  [unwired: 8 in, 1 out]
  n182 = Open VI Reference(type specifier VI Refnum (for type only)=refnum<vi> refnum, vi path=w40, options=128 ("选项")) -> (vi reference=w38:refnum<vi>, error out=w36:errorcluster)  [unwired: 3 in]
  n183 = vi-ref "氨氮断电保存全局变量.vi"() -> (w8:refnum<vi>)
  n184 = call-by-ref "?"(reference=w38, error in=w36) -> (reference out=w34:refnum<vi>, error out=w35:errorcluster)  [unwired: 12 in]
  n185 = Open VI Reference(type specifier VI Refnum (for type only)=refnum<vi> refnum, vi path=w26, options=128 ("选项")) -> (vi reference=w28:refnum<vi>, error out=w30:errorcluster)  [unwired: 3 in]
  n186 = call <userlib>:"Read Panel from INI__ogtk.vi"("error in (no error)"=w10, "VI ref"=w8, "refnum"=w7) -> ("error out"=w11:errorcluster, "refnum out"=w9:T18)  [unwired: 7 in]
  n187 = call-by-ref "?"(reference=w28, error in=w30) -> (reference out=w32:refnum<vi>, error out=w31:errorcluster)  [unwired: 12 in]
  n188 = Close Reference(reference=w34, error in (no error)=w35) -> ()  [unwired: 1 out]
  n189 = property on="曲线模型" class="氨氮曲线模型 (严格)"("属性"="氨氮" ("调用模块名称属性")) -> (error out=w2:errorcluster)  [unwired: 2 in, 1 out]
  n190 = Close Reference(reference=w32, error in (no error)=w31) -> ()  [unwired: 1 out]
  n191 = call <vilib>:"Close Config Data.vi"("error in (no error)"=w11, "refnum"=w9) -> ("error out"=w3:errorcluster)  [unwired: 8 in, 1 out]
  n192 = Obtain Notifier(name (unnamed)="NH3N" ("名称（未命名）"), notification data type=FALSE) -> (notifier out=w12:refnum<notifier>)  [unwired: 2 in, 2 out]
  n193 = Obtain Queue(name (unnamed)="NH3N" ("名称（未命名）"), element data type=cluster{"命令":string, "data":variant} {"命令"="", "data"=variant}) -> (queue out=w42:refnum<queue>, error out=w43:errorcluster)  [unwired: 3 in, 1 out]
  n194 = control-ref of="测量模式下拉列表"() -> (w22:refnum<vi>)
  n195 = control-ref of="量程切换阈值"() -> (w20:refnum<vi>)
  n196 = control-ref of="参数下拉列表"() -> (w23:refnum<vi>)
  n197 = control-ref of="量程下拉列表"() -> (w24:refnum<vi>)
  n198 = control-ref of="备用系数"() -> (w19:refnum<vi>)
  n199 = control-ref of="公式"() -> (w21:refnum<vi>)
  n200 = while {
    tunnel: w42 -> [w395]
    tunnel: w43 -> [_]
    shift-right: [w389] -> _
    shift-left: enum16{"氨氮", "总磷"}."氨氮" ("枚举") -> [w390]
    stop <- FALSE stop-if-true
    w388 = u16 3 items=["总磷"=1, "氨氮"=3] ("站号")
    # "试剂填充 172 \n管路清洗108\n氨氮92\n总磷131\n总磷海水147\n总氮76\n总氮海水92"
    n201 = Wait (ms)(milliseconds to wait=u32 1000 ("等待时间（毫秒）")) -> ()  [unwired: 1 out]
    n202 = global read "氨氮断电保存全局变量.vi" "流程文件路径"() -> (w377:path)
    n203 = global read "VAR氨氮全局变量.vi" "状态告警区"() -> (w386:T4)
    n204 = Bundle By Name(cluster=cluster{"命令":string, "data":variant} {"命令"="", "data"=variant} ("元素"), "命令"="读状态告警区", "data"=w388) -> (w397:cluster{"命令":string, "data":variant})
    n205 = local write "流程文件路径"(w377) -> ()
    n206 = Bundle By Name(cluster=cluster{"命令":string, "data":variant} {"命令"="", "data"=variant} ("元素"), "命令"="读测量数据区", "data"=w388) -> (w393:cluster{"命令":string, "data":variant})
    n207 = Unbundle By Name(w386) -> ("系统时间"=w385:timestamp)
    n208 = Enqueue Element(queue=w395, element=w397) -> (queue out=w391:refnum<queue>)  [unwired: 2 in, 2 out]
    n209 = Enqueue Element(queue=w391, element=w393) -> (queue out=w387:refnum<queue>)  [unwired: 2 in, 2 out]
    n210 = Get Date/Time In Seconds() -> (seconds since 1Jan1904=w384:timestamp)
    n211 = Subtract(x=w384, y=w385) -> (x-y=w383:dbl)
    n212 = Absolute Value(x=w383) -> (abs(x)=w382:dbl)
    n213 = global read "VAR氨氮全局变量.vi" "通讯状态"() -> (w378:bool)
    n214 = Greater Or Equal?(x=w382, y=120.0) -> (x >= y?=w380:bool)
    n215 = And(x=w378, y=w380) -> (x .and. y?=w379:bool)
    n216 = case shown="真" w379 {
      tunnel: w387 -> [_ w402]
      frame False {
      }
      frame True {
        n217 = call "氨氮启动命令.vi"("参数"=T19 {"站号"=3, "量程切换"=enum."AUTO", "控制命令"=enum."校时", "模式设置"=enum."待机", "测量间隔"=0}) -> ("启动命令"=w401:cluster{"命令":string, "data":variant})  [unwired: 10 in]
        n218 = Enqueue Element(queue=w402, element=w401) -> ()  [unwired: 2 in, 3 out]
      }
    }
    n219 = Increment(x=w390) -> (x+1=w389:enum16{"氨氮", "总磷"})
  }
  n220 = while {
    tunnel: w42 -> [w411]
    tunnel: w24 -> [w410]
    tunnel: w23 -> [w409]
    tunnel: w22 -> [w408]
    tunnel: w21 -> [w407]
    tunnel: w20 -> [w406]
    tunnel: w19 -> [w405]
    tunnel: w12 -> [w404]
    tunnel: w3 -> [_]
    tunnel: w2 -> [_]
    stop <- FALSE stop-if-true
    n221 = event shown="[9] \"手动启动\": 值改变" {
      selector: _ -> [_ _ _ _ _ _ _ _ _ _ _ _ _ _ _ _ _ _ _ _ _ _]
      dyn-events: _ -> [_ _ _ _ _ _ _ _ _ _ _ _ _ _ _ _ _ _ _ _ _ _]
      timeout: _ -> [_ _ _ _ _ _ _ _ _ _ _ _ _ _ _ _ _ _ _ _ _ _]
      tunnel: w411 -> [_ w419 w448 _ _ _ _ _ _ w515 _ w540 w545 _ _ _ _ _ _ _ _ _]
      tunnel: w410 -> [_ _ _ _ _ _ _ _ _ _ _ _ _ _ _ _ w561 _ w581 w590 w597 w608]
      tunnel: w409 -> [_ _ _ _ _ _ _ _ _ _ _ _ _ _ _ _ w559 _ w579 w592 w604 w615]
      tunnel: w408 -> [_ _ _ _ _ _ _ _ _ _ _ _ _ _ _ _ w560 _ w580 w591 w598 w610]
      tunnel: w407 -> [_ _ _ _ _ _ _ _ _ _ _ _ _ _ _ _ w555 _ _ _ _ _]
      tunnel: w406 -> [_ _ _ _ _ _ _ _ _ _ _ _ _ _ _ _ _ _ w575 _ _ _]
      tunnel: w405 -> [_ _ _ _ _ _ _ _ _ _ _ _ _ _ _ _ _ _ _ _ w602 _]
      tunnel: w404 -> [_ _ _ _ _ _ _ _ _ _ _ _ w543 _ _ _ _ _ _ _ _ _]
      event Timeout {
        n222 = event-data() -> ()  [unwired: 1 in, 3 out]
      }
      event "串口设置": Value Change {
        n223 = event-data() -> ()  [unwired: 1 in, 6 out]
        n224 = global read "氨氮断电保存全局变量.vi" "MB通信方式选择"() -> (w413:enum16{"串口", "TCP"})
        n225 = global read "氨氮断电保存全局变量.vi" "VISA Resource"() -> (w422:refnum<visa-resource-name>)
        n226 = global read "氨氮断电保存全局变量.vi" "PORT"() -> (w417:string)
        n227 = global read "氨氮断电保存全局变量.vi" "IP"() -> (w418:string)
        n228 = call "串口配置.vi"("PORT"=w417, "IP"=w418, "MB通信方式选择"=w413, "请选择串口:"=w422) -> ("PORT 2"=w415:string, "IP 2"=w416:string, "确认 2"=w421:bool, "VISA资源名称 2"=w420:refnum<visa-resource-name>, "MB通信方式选择 2"=w414:enum16{"串口", "TCP"})  [unwired: 3 in]
        n229 = case shown="真" w421 {
          tunnel: w420 -> [_ w427]
          tunnel: w419 -> [_ w426]
          tunnel: w416 -> [_ w425]
          tunnel: w415 -> [_ w424]
          tunnel: w414 -> [_ w423]
          frame False {
          }
          frame True {
            n230 = flat-sequence {
              tunnel: w427 -> [w433]
              tunnel: w426 -> [w431]
              tunnel: w425 -> [w430]
              tunnel: w424 -> [w429]
              tunnel: w423 -> [w428]
              frame #0 {
                n231 = global write "氨氮断电保存全局变量.vi" "IP"(w430) -> ()
                n232 = global write "氨氮断电保存全局变量.vi" "PORT"(w429) -> ()
                n233 = global write "氨氮断电保存全局变量.vi" "VISA Resource"(w433) -> ()
                n234 = global write "氨氮断电保存全局变量.vi" "MB通信方式选择"(w428) -> ()
                n235 = Enqueue Element(queue=w431, element=cluster{"命令":string, "data":variant} {"命令"="启用模块", "data"=variant} ("元素")) -> ()  [unwired: 2 in, 3 out]
              }
              frame #1 {
                n236 = call <vilib>:"Application Directory.vi"() -> ("Application Directory"=w447:path)
                n237 = Build Path(base path=w447, name or relative path="data\\sys.ini" ("名称或相对路径")) -> (appended path=w445:path)
                n238 = call <vilib>:"Open Config Data.vi"("configuration file path"=w445) -> ("error out"=w441:errorcluster, "refnum"=w444:T18)  [unwired: 8 in, 1 out]
                n239 = vi-ref "氨氮断电保存全局变量.vi"() -> (w443:refnum<vi>)
                n240 = call <userlib>:"Write Panel to INI__ogtk.vi"("error in (no error)"=w441, "VI ref"=w443, "refnum"=w444) -> ("error out"=w440:errorcluster, "refnum out"=w442:T18)  [unwired: 7 in]
                n241 = call <vilib>:"Close Config Data.vi"("error in (no error)"=w440, "refnum"=w442) -> ("error out"=w435:errorcluster, "file path"=w434:path)  [unwired: 8 in]
                n242 = Open/Create/Replace File(file path (use dialog)=w434, error in=w435) -> (refnum out=w438:refnum<file>, error out=w439:errorcluster)  [unwired: 4 in, 1 out]
                n243 = Flush File(refnum=w438, error in=w439) -> (refnum out=w437:refnum<file>, error out=w436:errorcluster)
                n244 = Close File(refnum=w437, error in=w436) -> ()  [unwired: 2 out]
              }
            }
          }
        }
      }
      event "模块启用": Value Change {
        n245 = event-data() -> ("OldVal"=w449:bool)  [unwired: 1 in, 5 out]
        n246 = case shown="假" w449 {
          tunnel: w448 -> [w450 w452]
          frame False {
            n247 = Enqueue Element(queue=w450, element=cluster{"命令":string, "data":variant} {"命令"="停用模块", "data"=variant} ("元素")) -> ()  [unwired: 2 in, 3 out]
          }
          frame True {
            n248 = Enqueue Element(queue=w452, element=cluster{"命令":string, "data":variant} {"命令"="启用模块", "data"=variant} ("元素")) -> ()  [unwired: 2 in, 3 out]
          }
        }
      }
      event "流程文件路径": Value Change {
        n249 = event-data() -> ()  [unwired: 1 in, 6 out]
        n250 = flat-sequence {
          frame #0 {
            n251 = local read "流程文件路径"() -> (w454:path)
            n252 = global write "氨氮断电保存全局变量.vi" "流程文件路径"(w454) -> ()
          }
          frame #1 {
            n253 = call <vilib>:"Application Directory.vi"() -> ("Application Directory"=w468:path)
            n254 = Build Path(base path=w468, name or relative path="data\\sys.ini" ("名称或相对路径")) -> (appended path=w466:path)
            n255 = call <vilib>:"Open Config Data.vi"("configuration file path"=w466) -> ("error out"=w462:errorcluster, "refnum"=w465:T18)  [unwired: 8 in, 1 out]
            n256 = vi-ref "氨氮断电保存全局变量.vi"() -> (w464:refnum<vi>)
            n257 = call <userlib>:"Write Panel to INI__ogtk.vi"("error in (no error)"=w462, "VI ref"=w464, "refnum"=w465) -> ("error out"=w461:errorcluster, "refnum out"=w463:T18)  [unwired: 7 in]
            n258 = call <vilib>:"Close Config Data.vi"("error in (no error)"=w461, "refnum"=w463) -> ("error out"=w456:errorcluster, "file path"=w455:path)  [unwired: 8 in]
            n259 = Open/Create/Replace File(file path (use dialog)=w455, error in=w456) -> (refnum out=w459:refnum<file>, error out=w460:errorcluster)  [unwired: 4 in, 1 out]
            n260 = Flush File(refnum=w459, error in=w460) -> (refnum out=w458:refnum<file>, error out=w457:errorcluster)
            n261 = Close File(refnum=w458, error in=w457) -> ()  [unwired: 2 out]
          }
        }
      }
      event "公式一键写入": Value Change {
        n262 = event-data() -> ()  [unwired: 1 in, 6 out]
        n263 = local read "公式"() -> (w469:cluster{"X^2":dbl, "X":dbl, "b":dbl})
        n264 = call "公式复合写入.vi"("公式"=w469) -> ()  [unwired: 11 in]
      }
      event "备用系数一键写入": Value Change {
        n265 = event-data() -> ()  [unwired: 1 in, 6 out]
        n266 = local read "备用系数"() -> (w470:T2)
        n267 = call "量程参数复合参数写入.vi"("备用系数"=w470) -> ()  [unwired: 11 in]
      }
      event "曲线模型": Value Change {
        n268 = event-data() -> ()  [unwired: 1 in, 6 out]
        n269 = local write "公式"("曲线模型") -> ()
      }
      event "质控参数设置": Value Change {
        n270 = event-data() -> ()  [unwired: 1 in, 6 out]
        n271 = global read "氨氮断电保存全局变量.vi" "质控参数设置"() -> (w472:T20)
        n272 = call "质控参数设置.vi"("质控参数设置"=w472) -> ("输出簇"=w473:T21)  [unwired: 10 in]
        n273 = Unbundle By Name(w473) -> ("确定"=w474:bool)
        n274 = case shown="真" w474 {
          tunnel: w473 -> [_ w476]
          tunnel: w472 -> [_ w475]
          frame False {
          }
          frame True {
            n275 = flat-sequence {
              tunnel: w476 -> [w483]
              tunnel: w475 -> [w477]
              frame #0 {
                n276 = Unbundle By Name(w483) -> ("跨度值"=w482:dbl, "零点标准液浓度"=w481:dbl, "跨度标准液浓度"=w480:dbl, "标准液标准浓度"=w479:dbl)
                n277 = Bundle By Name(cluster=w477, "跨度值"=w482, "零点标准液浓度"=w481, "跨度标准液浓度"=w480, "标准液标准浓度"=w479) -> (w478:T20)
                n278 = global write "氨氮断电保存全局变量.vi" "质控参数设置"(w478) -> ()
              }
              frame #1 {
                n279 = call <vilib>:"Application Directory.vi"() -> ("Application Directory"=w484:path)
                n280 = Build Path(base path=w484, name or relative path="data\\sys.ini" ("名称或相对路径")) -> (appended path=w486:path)
                n281 = call <vilib>:"Open Config Data.vi"("configuration file path"=w486) -> ("error out"=w490:errorcluster, "refnum"=w487:T18)  [unwired: 8 in, 1 out]
                n282 = vi-ref "氨氮断电保存全局变量.vi"() -> (w488:refnum<vi>)
                n283 = call <userlib>:"Write Panel to INI__ogtk.vi"("error in (no error)"=w490, "VI ref"=w488, "refnum"=w487) -> ("error out"=w491:errorcluster, "refnum out"=w489:T18)  [unwired: 7 in]
                n284 = call <vilib>:"Close Config Data.vi"("error in (no error)"=w491, "refnum"=w489) -> ("error out"=w496:errorcluster, "file path"=w497:path)  [unwired: 8 in]
                n285 = Open/Create/Replace File(file path (use dialog)=w497, error in=w496) -> (refnum out=w493:refnum<file>, error out=w492:errorcluster)  [unwired: 4 in, 1 out]
                n286 = Flush File(refnum=w493, error in=w492) -> (refnum out=w494:refnum<file>, error out=w495:errorcluster)
                n287 = Close File(refnum=w494, error in=w495) -> ()  [unwired: 2 out]
              }
            }
          }
        }
      }
      event "氨氮自动测试量程配置": Value Change {
        n288 = event-data() -> ()  [unwired: 1 in, 6 out]
        n289 = flat-sequence {
          frame #0 {
            n290 = global write "氨氮断电保存全局变量.vi" "氨氮自动测试量程配置"("氨氮自动测试量程配置") -> ()
          }
          frame #1 {
            n291 = call <vilib>:"Application Directory.vi"() -> ("Application Directory"=w512:path)
            n292 = Build Path(base path=w512, name or relative path="data\\sys.ini" ("名称或相对路径")) -> (appended path=w510:path)
            n293 = call <vilib>:"Open Config Data.vi"("configuration file path"=w510) -> ("error out"=w506:errorcluster, "refnum"=w509:T18)  [unwired: 8 in, 1 out]
            n294 = vi-ref "氨氮断电保存全局变量.vi"() -> (w508:refnum<vi>)
            n295 = call <userlib>:"Write Panel to INI__ogtk.vi"("error in (no error)"=w506, "VI ref"=w508, "refnum"=w509) -> ("error out"=w505:errorcluster, "refnum out"=w507:T18)  [unwired: 7 in]
            n296 = call <vilib>:"Close Config Data.vi"("error in (no error)"=w505, "refnum"=w507) -> ("error out"=w500:errorcluster, "file path"=w499:path)  [unwired: 8 in]
            n297 = Open/Create/Replace File(file path (use dialog)=w499, error in=w500) -> (refnum out=w503:refnum<file>, error out=w504:errorcluster)  [unwired: 4 in, 1 out]
            n298 = Flush File(refnum=w503, error in=w504) -> (refnum out=w502:refnum<file>, error out=w501:errorcluster)
            n299 = Close File(refnum=w502, error in=w501) -> ()  [unwired: 2 out]
          }
        }
      }
      event "手动启动": Value Change {
        n300 = event-data() -> ()  [unwired: 1 in, 6 out]
        n301 = call "氨氮启动参数对话框.vi"() -> ("确认"=w513:bool, "元素"=w514:cluster{"命令":string, "data":variant})  [unwired: 10 in]
        n302 = case shown="真" w513 {
          tunnel: w515 -> [_ w517]
          tunnel: w514 -> [_ w516]
          frame False {
          }
          frame True {
            n303 = Enqueue Element(queue=w517, element=w516) -> ()  [unwired: 2 in, 3 out]
          }
        }
      }
      event "定时启动": Mouse Down {
        n304 = event-data() -> ()  [unwired: 1 in, 6 out]
        n305 = flat-sequence {
          frame #0 {
            n306 = global read "氨氮断电保存全局变量.vi" "定时控制"() -> (w518:T6)
            n307 = call "周期设置.vi"("定时控制输入"=w518) -> ("定时控制输出"=w519:T6)  [unwired: 10 in]
            n308 = global write "氨氮断电保存全局变量.vi" "定时控制"(w519) -> ()
          }
          frame #1 {
            n309 = call <vilib>:"Application Directory.vi"() -> ("Application Directory"=w533:path)
            n310 = Build Path(base path=w533, name or relative path="data\\sys.ini" ("名称或相对路径")) -> (appended path=w531:path)
            n311 = call <vilib>:"Open Config Data.vi"("configuration file path"=w531) -> ("error out"=w527:errorcluster, "refnum"=w530:T18)  [unwired: 8 in, 1 out]
            n312 = vi-ref "氨氮断电保存全局变量.vi"() -> (w529:refnum<vi>)
            n313 = call <userlib>:"Write Panel to INI__ogtk.vi"("error in (no error)"=w527, "VI ref"=w529, "refnum"=w530) -> ("error out"=w526:errorcluster, "refnum out"=w528:T18)  [unwired: 7 in]
            n314 = call <vilib>:"Close Config Data.vi"("error in (no error)"=w526, "refnum"=w528) -> ("error out"=w521:errorcluster, "file path"=w520:path)  [unwired: 8 in]
            n315 = Open/Create/Replace File(file path (use dialog)=w520, error in=w521) -> (refnum out=w524:refnum<file>, error out=w525:errorcluster)  [unwired: 4 in, 1 out]
            n316 = Flush File(refnum=w524, error in=w525) -> (refnum out=w523:refnum<file>, error out=w522:errorcluster)
            n317 = Close File(refnum=w523, error in=w522) -> ()  [unwired: 2 out]
          }
        }
      }
      event "单步测试": Value Change {
        w535 = u16 1 items=["总磷"=1, "氨氮"=3] ("站号")
        n318 = event-data() -> ()  [unwired: 1 in, 6 out]
        n319 = Bundle("站号"=w535, "总磷氨氮调试"="总磷氨氮调试") -> (w534:cluster{"站号":u16, "总磷氨氮调试":u16[]})  [unwired: 1 in]
        n320 = Bundle By Name(cluster=cluster{"命令":string, "data":variant} {"命令"="", "data"=variant} ("元素"), "命令"="debug", "data"=w534) -> (w537:cluster{"命令":string, "data":variant})
        n321 = Enqueue Element(queue=w540, element=w537) -> ()  [unwired: 2 in, 3 out]
      }
      event "停止": Value Change {
        n322 = event-data() -> ()  [unwired: 1 in, 6 out]
        n323 = Enqueue Element(queue=w545, element=cluster{"命令":string, "data":variant} {"命令"="启动", "data"=variant(cluster{"站号":u16, "控制命令输出":u16[]} {"站号"=3, "控制命令输出"=[2816]})} ("启动命令")) -> ()  [unwired: 2 in, 3 out]
        n324 = Cancel Notification(0:w543) -> (8:w542:refnum<notifier>)  [unwired: 1 in, 2 out]
        n325 = Send Notification(notification=TRUE ("通知"), notifier=w542) -> ()  [unwired: 1 in, 2 out]
      }
      event "设置": Value Change {
        n326 = event-data() -> ()  [unwired: 1 in, 6 out]
        n327 = property on="窗格" class="Pane"("Origin"=T10 {"Horizontal"=0, "Vertical"=628} ("原点")) -> ()  [unwired: 2 in, 2 out]
      }
      event "返回": Value Change {
        n328 = event-data() -> ()  [unwired: 1 in, 6 out]
        n329 = property on="窗格" class="Pane"("Origin"=T10 {"Horizontal"=0, "Vertical"=0} ("原点")) -> ()  [unwired: 2 in, 2 out]
      }
      event "公式.X^2", "公式.X", "公式.b", "量程切换阈值.阈值", "量程切换阈值.标液浓度", "备用系数.量程上限", "备用系数.量程下限", "备用系数.检出限", "备用系数.精度": Mouse Down {
        n330 = event-data() -> ("CtlRef"=w551:refnum<vi>)  [unwired: 1 in, 5 out]
        n331 = property class="DigNum (严格)"(reference=w551) -> (reference out=w549:refnum<vi>, "Value"=w550:dbl)  [unwired: 1 in, 1 out]
        n332 = call "数字键盘.vi"("OldNumber"=w550) -> ("NewNumber"=w548:dbl)
        n333 = property class="DigNum (严格)"(reference=w549, "Val(Sgnl)"=w548) -> ()  [unwired: 1 in, 2 out]
      }
      event "读公式": Value Change {
        n334 = event-data() -> ()  [unwired: 1 in, 6 out]
        n335 = property class="Enum (严格)"(reference=w559) -> ("Value"=w558:enum16{"氨氮", "总磷"})  [unwired: 1 in, 2 out]
        n336 = property class="Enum (严格)"(reference=w560) -> ("Value"=w557:enum16{"水样测量", "空白核查", "跨度核查", "标样核查", "加标回收"})  [unwired: 1 in, 2 out]
        n337 = property class="Enum (严格)"(reference=w561) -> ("Value"=w556:enum16{"低量程", "高量程"})  [unwired: 1 in, 2 out]
        n338 = call "氨氮公式读取.vi"("量程"=w556, "测量模式"=w557, "测量参数"=w558) -> ("error out"=w553:errorcluster, "公式"=w554:cluster{"X^2":dbl, "X":dbl, "b":dbl})  [unwired: 7 in]
        n339 = property class="Clust (严格)"(reference=w555, "Value"=w554) -> ()  [unwired: 1 in, 2 out]
        n340 = case shown="错误" w553 {
          tunnel: ["读取成功" ("消息") "读取失败" ("消息")] -> w552
          frame No Error {
          }
          frame Error {
          }
        }
        n341 = One Button Dialog(message=w552) -> ()  [unwired: 1 in, 1 out]
      }
      event "写公式": Value Change {
        n342 = event-data() -> ()  [unwired: 1 in, 6 out]
        n343 = call "氨氮公式写入.vi"("公式"="公式", "量程"="量程下拉列表", "测量模式"="测量模式下拉列表", "测量参数"="参数下拉列表") -> ("error out"=w564:errorcluster)  [unwired: 7 in]
        n344 = case shown="无错误" w564 {
          tunnel: ["写入成功" ("消息") "写入失败" ("消息")] -> w565
          frame No Error {
          }
          frame Error {
          }
        }
        n345 = One Button Dialog(message=w565) -> ()  [unwired: 1 in, 1 out]
      }
      event "量程切换阈值读取": Value Change {
        n346 = event-data() -> ()  [unwired: 1 in, 6 out]
        n347 = property class="Enum (严格)"(reference=w579) -> ("Value"=w578:enum16{"氨氮", "总磷"})  [unwired: 1 in, 2 out]
        n348 = property class="Enum (严格)"(reference=w580) -> ("Value"=w577:enum16{"水样测量", "空白核查", "跨度核查", "标样核查", "加标回收"})  [unwired: 1 in, 2 out]
        n349 = property class="Enum (严格)"(reference=w581) -> ("Value"=w576:enum16{"低量程", "高量程"})  [unwired: 1 in, 2 out]
        n350 = call "氨氮量程读取.vi"("量程"=w576, "测量模式"=w577, "测量参数"=w578) -> ("error out"=w572:errorcluster, "量程切换阈值"=w574:cluster{"阈值":dbl, "标液浓度":dbl})  [unwired: 7 in]
        n351 = property class="Clust (严格)"(reference=w575, "Value"=w574) -> ()  [unwired: 1 in, 2 out]
        n352 = case shown="错误" w572 {
          tunnel: ["读取成功" ("消息") "读取失败" ("消息")] -> w573
          frame No Error {
          }
          frame Error {
          }
        }
        n353 = One Button Dialog(message=w573) -> ()  [unwired: 1 in, 1 out]
      }
      event "量程切换阈值写入": Value Change {
        n354 = event-data() -> ()  [unwired: 1 in, 6 out]
        n355 = property class="Enum (严格)"(reference=w592) -> ("Value"=w589:enum16{"氨氮", "总磷"})  [unwired: 1 in, 2 out]
        n356 = property class="Enum (严格)"(reference=w591) -> ("Value"=w588:enum16{"水样测量", "空白核查", "跨度核查", "标样核查", "加标回收"})  [unwired: 1 in, 2 out]
        n357 = property class="Enum (严格)"(reference=w590) -> ("Value"=w587:enum16{"低量程", "高量程"})  [unwired: 1 in, 2 out]
        n358 = call "氨氮量程写入.vi"("量程切换阈值"="量程切换阈值", "量程"=w587, "测量模式"=w588, "测量参数"=w589) -> ("error out"=w584:errorcluster)  [unwired: 7 in]
        n359 = case shown="无错误" w584 {
          tunnel: ["写入成功" ("消息") "写入失败" ("消息")] -> w585
          frame No Error {
          }
          frame Error {
          }
        }
        n360 = One Button Dialog(message=w585) -> ()  [unwired: 1 in, 1 out]
      }
      event "备用系数读取": Value Change {
        n361 = event-data() -> ()  [unwired: 1 in, 6 out]
        n362 = property class="Enum (严格)"(reference=w604) -> ("Value"=w603:enum16{"氨氮", "总磷"})  [unwired: 1 in, 2 out]
        n363 = property class="Enum (严格)"(reference=w598) -> ("Value"=w595:enum16{"水样测量", "空白核查", "跨度核查", "标样核查", "加标回收"})  [unwired: 1 in, 2 out]
        n364 = property class="Enum (严格)"(reference=w597) -> ("Value"=w596:enum16{"低量程", "高量程"})  [unwired: 1 in, 2 out]
        n365 = call "氨氮备用系数读取.vi"("量程"=w596, "测量模式"=w595, "测量参数"=w603) -> ("error out"=w599:errorcluster, "备用系数"=w601:T2)  [unwired: 7 in]
        n366 = property class="Clust (严格)"(reference=w602, "Value"=w601) -> ()  [unwired: 1 in, 2 out]
        n367 = case shown="错误" w599 {
          tunnel: ["读取成功" ("消息") "读取失败" ("消息")] -> w600
          frame No Error {
          }
          frame Error {
          }
        }
        n368 = One Button Dialog(message=w600) -> ()  [unwired: 1 in, 1 out]
      }
      event "备用系数写入": Value Change {
        n369 = event-data() -> ()  [unwired: 1 in, 6 out]
        n370 = property class="Enum (严格)"(reference=w615) -> ("Value"=w614:enum16{"氨氮", "总磷"})  [unwired: 1 in, 2 out]
        n371 = property class="Enum (严格)"(reference=w610) -> ("Value"=w609:enum16{"水样测量", "空白核查", "跨度核查", "标样核查", "加标回收"})  [unwired: 1 in, 2 out]
        n372 = property class="Enum (严格)"(reference=w608) -> ("Value"=w607:enum16{"低量程", "高量程"})  [unwired: 1 in, 2 out]
        n373 = call "氨氮备用系数写入.vi"("备用系数"="备用系数", "量程"=w607, "测量模式"=w609, "测量参数"=w614) -> ("error out"=w611:errorcluster)  [unwired: 7 in]
        n374 = case shown="无错误" w611 {
          tunnel: ["写入成功" ("消息") "写入失败" ("消息")] -> w612
          frame No Error {
          }
          frame Error {
          }
        }
        n375 = One Button Dialog(message=w612) -> ()  [unwired: 1 in, 1 out]
      }
    }
  }
